vi "TEST_L1_COMPLETE.vi"() -> ()   [LabVIEW 2012]
uses:
  <vilib>/Utility/NIReport.llb/NI_report.lvclass
  <vilib>/Utility/NIReport.llb/HTML/NI_HTML.lvclass
  Sum_Abrilader/L0_Sum_Adder Folder/C/Program Files/National Instruments/LabVIEW 2012/instr.lib/Agilent 8000 Series/Public/Data/Low Level/Fetch Measurement (More).vi
  <instrlib>/Agilent 8000 Series/Agilent 8000 Series.lvlib
  Sum_Abrilader/L0_Sum_Adder Folder/C/Program Files/National Instruments/LabVIEW 2012/instr.lib/Agilent 81150/Agilent 81150.lvlib
panel:
  out "IPR_count":u32
  in  "step":i32=1
  in  "min DT":i32
  in  "max DT":dbl=90.0
  in  "Gains":dbl[](array[numeric])=[0.96, 0.97, 0.98, 0.88, 1.0, 1.0, 0.99]
  in  "Pulse Amplitude":dbl=0.3
  in  "Instrument VISA in":T1={"AWG VISA"="AgilentGenerator1", "Oscilloscope  VISA "="AgilentOsciloscope", "Integration Board IP"="172.16.17.48", "connection ID"=refnum, "report out"=refnum, "report file path"=path "C:/Users/omartinez/Desktop/L0nL1_Results"}
  out "data out serial":string="empty_read_bufferwrittingempty_read_bufferwritting2"
  in  "Combination\n  (Act High)":i32 min=0 max=127 step=1 format="%b"
  in  "Single/Comb":bool=TRUE
  in  "Single Channel Enable":i32(slide) scale=0.0..6.0
  out "error out":errorcluster
  in  "error in (no error)":errorcluster
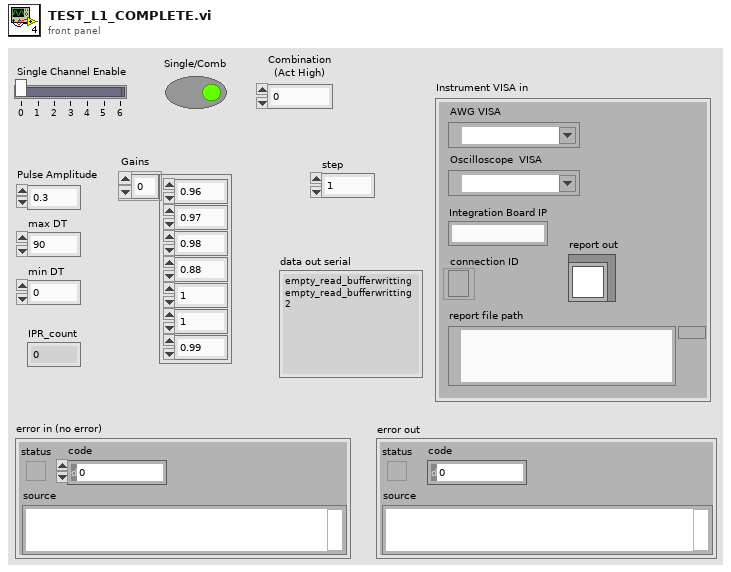
[diagram p1: front panel]
types:
  T1 = cluster{"AWG VISA":refnum<visa-resource-name>, "Oscilloscope  VISA ":refnum<visa-resource-name>, "Integration Board IP":string, "connection ID":refnum<k5>, "report out":refnum<class "NI_report.lvclass">, "report file path":path}
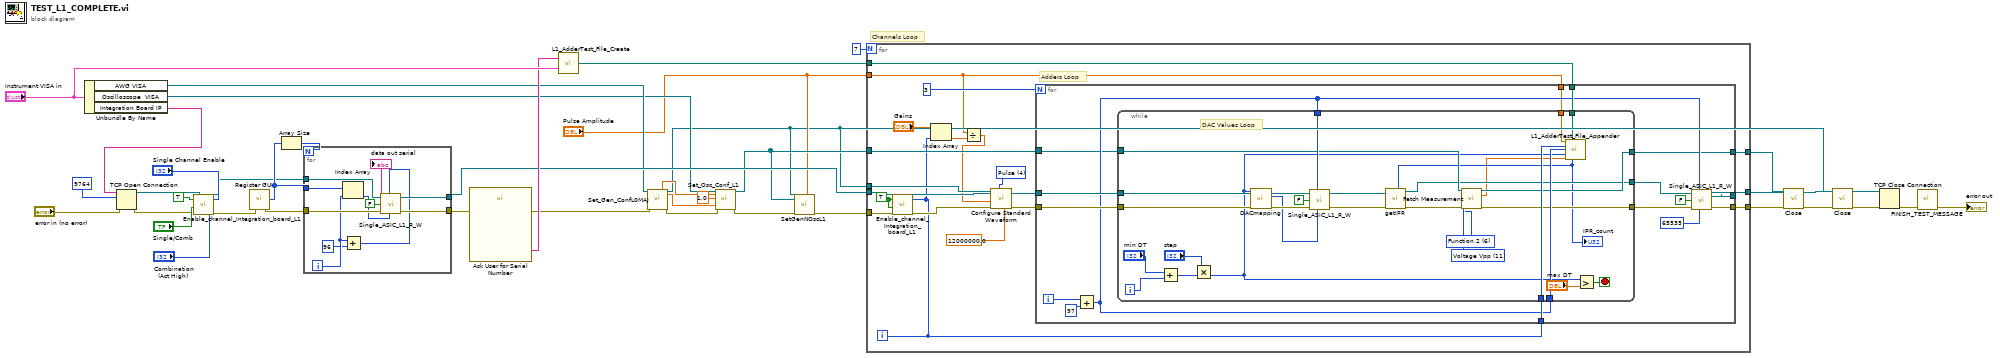
[diagram p0: block diagram]
diagram:
  # "Channels Loop"
  n1 = Unbundle By Name("Instrument VISA in") -> ("AWG VISA"=w14:refnum<visa-resource-name>, "Oscilloscope  VISA"=w13:refnum<visa-resource-name>, "Integration Board IP"=w24:string)
  n2 = TCP Open Connection(address=w24, remote port or service name=9764, error in (no error)="error in (no error)") -> (connection ID=w31:refnum<k5>, error out=w32:errorcluster)  [unwired: 2 in]
  n3 = call "Enable_channel_Integration_board_L1.vi"("Cobination"="Combination\n  (Act High)", "Enable  L1 single  Input"="Single Channel Enable", "error in (no error)"=w32, "SingleIN/#Combination"="Single/Comb", "#Enable all L1"=TRUE, "connection ID"=w31) -> ("error out"=w25:errorcluster, "connection ID out"=w27:refnum<k5>)
  n4 = call "Register GUI.vi"("error in (no error)"=w25) -> ("error out"=w30:errorcluster, "REG ARRAy"=w28:u32[])  [unwired: 3 in]
  n5 = Array Size(array=w28) -> (size(s)=w29:i32)
  n6 = for {
    N: w29 -> [_]
    tunnel: w30 -> [w50]
    tunnel: w28 -> [w49]
    tunnel: w27 -> [w48]
    tunnel: [w47] -> w18
    tunnel: [w46] -> w21
    i -> [w42]
    n7 = Index Array(array=w49, index=w42) -> (element=w45:u32)
    n8 = Add(x=w42, y=96) -> (x+y=w43:i32)
    n9 = call "Single_ASIC_L1_R_W.vi"("connection ID"=w48, "Register or channel"=w43, "RD/#WR"=FALSE, "error in (no error)"=w50, "Data"=w45) -> ("data out serial"=→"data out serial":string, "connection ID out"=w47:refnum<k5>, "error out"=w46:errorcluster)  [unwired: 1 in, 1 out]
  }
  n10 = call "Ask User for Serial Number"("error in (no error)"=w21) -> ("Serial Number"=w20:string, "error out"=w12:errorcluster)  [unwired: 16 in, 1 out]
  n11 = call "L1_AdderTest_File_Create.vi"("input cluster"="Instrument VISA in", "Serial Number"=w20) -> ("appended path"=w19:path)
  n12 = call "Set_Gen_ConfL0MAJ.vi"("AWG VISA"=w14, "error in (no error)"=w12) -> ("Amplitude 1 OUT"=w16:dbl, "VISA resource name out"=w2:refnum<visa-resource-name>, "Pulse Width in seconds 1 OUT"=w15:dbl, "error out"=w17:errorcluster)  [unwired: 10 in, 4 out]
  n13 = call "Set_Osc_Conf_L1.vi"("VISA resource name"=w13, "Amplitude IN"=w16, "Trigger Level IN"=1.0, "Pulse Width in seconds IN"=w15, "error in (no error)"=w17) -> ("VISA resource name out"=w5:refnum<visa-resource-name>, "error out"=w7:errorcluster)  [unwired: 13 in]
  n14 = call "SetGenNOscL1.vi"("Input Voltage"="Pulse Amplitude", "error in (no error)"=w7, "VISA resource name"=w5, "AWG VISA"=w2) -> ("error out 2"=w6:errorcluster)  [unwired: 7 in]
  n15 = for {
    N: 7 -> [_]
    tunnel: [w70] -> w11
    tunnel: [w68] -> w26
    tunnel: w18 -> [w66]
    tunnel: w19 -> [w64]
    tunnel: "Pulse Amplitude" -> [w55]
    tunnel: w6 -> [w63]
    tunnel: w5 -> [w62]
    tunnel: [w61] -> w8
    tunnel: w2 -> [w57]
    i -> [w56]
    w60 = u16 4 items=["Sine", "Square", "Ramp Up", "Ramp Down", "Pulse", "Noise", "DC"] ("Waveform (0: Sine)")
    w65 = TRUE ("#Enable all L1")
    # "Adders Loop"
    n16 = call "Enable_channel_Integration_board_L1.vi"("Enable  L1 single  Input"=w56, "error in (no error)"=w63, "SingleIN/#Combination"=w65, "#Enable all L1"=w65, "connection ID"=w66) -> ("error out"=w59:errorcluster, "connection ID out"=w67:refnum<k5>)  [unwired: 1 in]
    n17 = Index Array(array="Gains", index=w56) -> (element=w54:dbl)
    n18 = Divide(x=w55, y=w54) -> (x/y=w53:dbl)
    n19 = call <instrlib>:"Configure Standard Waveform.vi"("Frequency (1000.0 Hz)"=12000000.0, "Waveform (0: Sine)"=w60, "error in (no error)"=w59, "Amplitude (1.0 Vpp)"=w53, "VISA resource name"=w57) -> ("error out"=w58:errorcluster)  [unwired: 5 in, 1 out]
    n20 = for {
      N: 3 -> [_]
      tunnel: w67 -> [w86]
      tunnel: w58 -> [w83]
      tunnel: [w82] -> w70
      tunnel: [w80] -> w68
      tunnel: w64 -> [w77]
      tunnel: w56 -> [w76]
      tunnel: w55 -> [w74]
      tunnel: w62 -> [w72]
      tunnel: [w71] -> w61
      i -> [w84]
      n21 = Add(x=w84, y=97) -> (x+y=w75:i32)
      n22 = while {
        tunnel: w86 -> [w114]
        tunnel: w75 -> [w112]
        tunnel: w83 -> [w111]
        tunnel: [w95] -> w81
        tunnel: [w101] -> w73
        tunnel: w77 -> [w107]
        tunnel: w76 -> [w106]
        tunnel: w75 -> [w105]
        tunnel: w74 -> [w104]
        tunnel: w72 -> [w100]
        tunnel: [w99] -> w71
        i -> [w89]
        stop <- w108 stop-if-true
        w103 = 11 items=["Rise Time", "Fall Time", "Frequency", "Period", "Voltage RMS(AC)", "Voltage RMS(DC)", "Voltage RMS (AC,cycle)", "Voltage RMS (DC,cycle)", "Voltage Max", "Voltage Min", "Voltage Middle", "Voltage Vpp", "Voltage High", "Voltage Low", "Voltage Average", "Voltage Average (cycle)", "Width Negative", "Width Positive", "Duty Cycle Positive", "Amplitude", "Overshoot", "Preshoot", "Voltage Base", "Voltage Upper", "Time Max", "Time Min", "Color Grade Crossing", "Color Grade Eye Width", "Color Grade Eye Height", "Color Grade Eye Q-Factory", "Color Grade Eye Duty Cycle Distortion(Percent)", "Color Grade Eye Duty Cycle Distortion(Time)", "Color Grade Eye Jitter(PP)", "Color Grade Eye Width(RMS)", "Cycle-cycle Duty Jitter(Rising)", "Cycle-cycle Duty Jitter(Falling)", "Cycle-cycle Jitter(Rising)", "Cycle-cycle Jitter(Falling)", "Cycle-cycle - Width", "Cycle-cycle + Width", "Date Rate", "Unit Interval", "FFT Delta Frequency", "FFT Delta Magnitude", "FFT Frequency", "FFT Magnitude", "Slew Rate", "Area (Entire Display)", "Area(Single Cycle)", "Duty Cycle (Rising)", "Duty Cycle (Falling)"] ("Measurement Function (0: Rise Time)")
        w102 = 6 items=["Channel 1"=1, "Channel 2"=2, "Channel 3"=3, "Channel 4"=4, "Function 1"=5, "Function 2"=6, "Function 3"=7, "Function 4"=8, "Memory 1"=9, "Memory 2"=10, "Memory 3"=11, "Memory 4"=12] ("Channel (1: Channel 1)")
        # "DAC Values Loop"
        n23 = Add(x="min DT", y=w89) -> (x+y=w92:i32)
        n24 = Multiply(x="step", y=w92) -> (x*y=w88:i32)
        n25 = call "DACmapping.vi"("error in (no error)"=w111, "DAC_TH2"=w88) -> ("error out"=w110:errorcluster, "COMB DEC"=w109:u32)  [unwired: 8 in]
        n26 = call "Single_ASIC_L1_R_W.vi"("connection ID"=w114, "Register or channel"=w112, "RD/#WR"=FALSE, "error in (no error)"=w110, "Data"=w109) -> ("connection ID out"=w96:refnum<k5>, "error out"=w98:errorcluster)  [unwired: 1 in, 2 out]
        n27 = call "getIPR.vi"("error in"=w98, "connection ID"=w96) -> ("error out"=w97:errorcluster, "connection ID out"=w95:refnum<k5>, "IPR_count"=w94:u32)  [unwired: 6 in, 1 out]
        "IPR_count" <- w94
        n28 = call-poly "Fetch Measurement.vi"("VISA resource name"=w100, "Channel (1: Channel 1)"=w102, "Measurement Function (0: Rise Time)"=w103, "error in (no error)"=w97) -> ("VISA resource name out"=w99:refnum<visa-resource-name>, "Measurement"=w93:dbl, "error out"=w101:errorcluster)  [unwired: 9 in]
        n29 = call "L1_AdderTest_File_Appender.vi"("Vin"=w104, "file path (dialog if empty)"=w107, "CH"=w106, "Active Adder"=w105, "DAC Level"=w88, "Vmeas"=w93, "IPR"=w94) -> ()  [unwired: 9 in]
        n30 = Greater?(x=w88, y="max DT") -> (0:w108:bool)
      }
      n31 = call "Single_ASIC_L1_R_W.vi"("connection ID"=w81, "Register or channel"=w75, "RD/#WR"=FALSE, "error in (no error)"=w73, "Data"=u32 65535 ("COMB DEC")) -> ("connection ID out"=w80:refnum<k5>, "error out"=w82:errorcluster)  [unwired: 1 in, 2 out]
    }
  }
  n32 = call <instrlib>:"Close.vi"("error in (no error)"=w11, "VISA resource name"=w8) -> ("error out"=w10:errorcluster)  [unwired: 9 in]
  n33 = call <instrlib>:"Close.vi"("error in (no error)"=w10, "VISA resource name"=w2) -> ("error out"=w9:errorcluster)  [unwired: 9 in]
  n34 = TCP Close Connection(connection ID=w26, error in (no error)=w9) -> (error out=w37:errorcluster)  [unwired: 1 in, 1 out]
  n35 = call "FINISH_TEST_MESSAGE.vi"("error in"=w37) -> ("error out"=→"error out":errorcluster)  [unwired: 10 in]
